vi "Init Cubic Spline + Sine Parameters.vi"(6 "Weighted Fit":T3, 8 "error in (no error)":errorcluster, 9 "Cubic Spline + Sine Options":T1, 10 "Y axis in":dbl[](array[numeric]), 11 "t Axis in":dbl[](array[numeric])) -> (0 "error out":errorcluster, 1 "Cubic Spline + Sine Options":T1, 2 "Initial Parameters":dbl[](array[numeric]), 3 "Weights":dbl[](array[numeric]), 4 "parameter bounds":T2)   [LabVIEW 2021, in "Fits.lvlib"]
uses:
  Fits.lvlib
  Cubic Spline + Sine Options.ctl
  IRF(X)PSED/Fit Weights Type v2.ctl
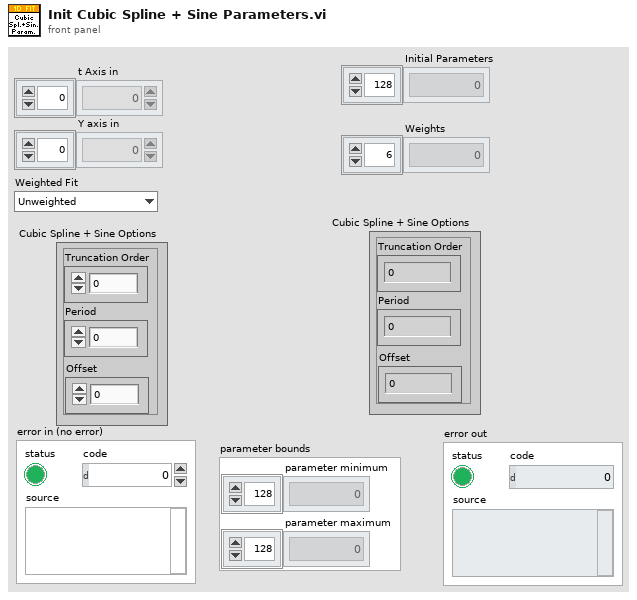
[diagram p1: front panel]
types:
  T1 = typedef "Fits.lvlib/Cubic Spline + Sine Options.ctl" = cluster{"Truncation Order":i32, "Period":dbl, "Offset":dbl}
  T2 = cluster{"parameter minimum":dbl[], "parameter maximum":dbl[]}
  T3 = typedef "Fits.lvlib/Fit Weights Type v2.ctl" = enum16{"Unweighted", "1/Variance (Neyman)", "1/Variance (Pearson)", "Best of All"}
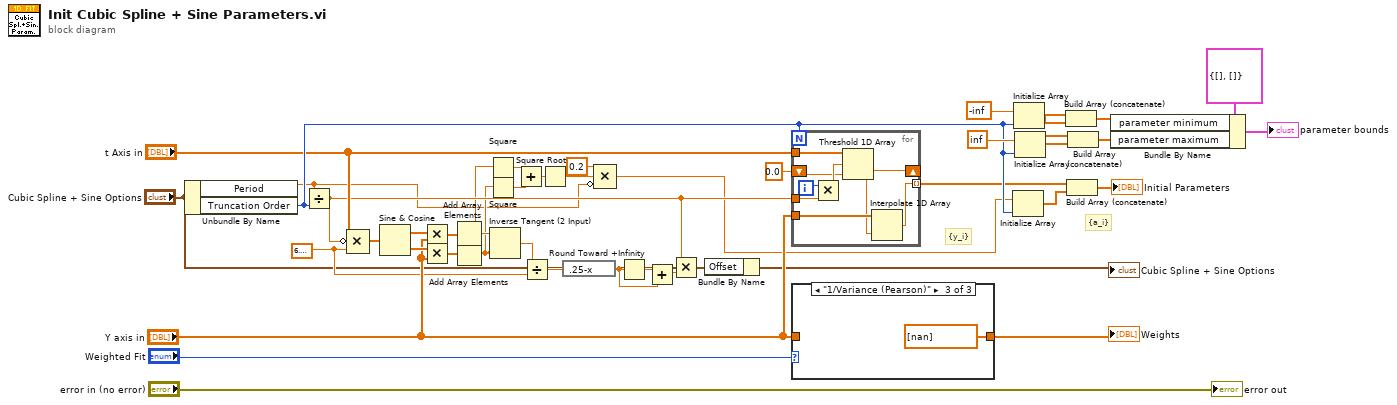
[diagram p0: block diagram]
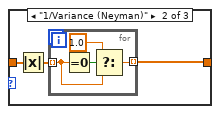
[diagram p3: hidden frame]
diagram:
  w18 = 6.283185307179586
  # "{a_i}"
  # "{y_i}"
  n1 = Unbundle By Name("Cubic Spline + Sine Options") -> ("Period"=w2:dbl, "Truncation Order"=w30:i32)
  n2 = Divide(x=w2, y=w30) -> (x/y=w13:dbl)
  n3 = Compound Arithmetic op=MULTIPLY("t Axis in", invert w13, w18) -> (w25:dbl[])
  n4 = Sine & Cosine(0:w25) -> (1:w23:dbl[], 2:w24:dbl[])
  n5 = Multiply(x=w23, y="Y axis in") -> (x*y=w21:dbl[])
  n6 = Multiply(x=w24, y="Y axis in") -> (x*y=w20:dbl[])
  n7 = Add Array Elements(numeric array=w21) -> (sum=w9:dbl)
  n8 = Add Array Elements(numeric array=w20) -> (sum=w8:dbl)
  n9 = Square(x=w9) -> (x^2=w7:dbl)
  n10 = Square(x=w8) -> (x^2=w6:dbl)
  n11 = Inverse Tangent (2 Input)(1:w8, 2:w9) -> (0:w19:dbl)
  n12 = Add(x=w7, y=w6) -> (x+y=w5:dbl)
  n13 = Divide(x=w19, y=w18) -> (x/y=w17:dbl)
  n14 = Square Root(x=w5) -> (sqrt(x)=w4:dbl)
  n15 = expression code=".25-x"(w17) -> (w15:dbl)
  n16 = Compound Arithmetic op=MULTIPLY(0.2 ("value"), w4, invert w2) -> (w1:dbl)
  n17 = Round Toward +Infinity(x=w15) -> (ceil(x): smallest int >= x=w16:dbl)
  n18 = Add(x=w16, y=w15) -> (x+y=w14:dbl)
  n19 = Multiply(x=w13, y=w14) -> (x*y=w11:dbl)
  n20 = Bundle By Name(cluster="Cubic Spline + Sine Options", "Offset"=w11) -> (→"Cubic Spline + Sine Options":T1)
  n21 = for {
    N: w30 -> [_]
    tunnel: "Y axis in" -> [w50]
    tunnel: [w49] -> w28 mode=indexing
    tunnel: w13 -> [w48]
    tunnel: "t Axis in" -> [w46]
    shift-right: [w43] -> _
    shift-left: 0.0 -> [w44]
    i -> [w47]
    n22 = Multiply(x=w47, y=w48) -> (x*y=w45:dbl)
    n23 = Threshold 1D Array(1:w44, 2:w45, 3:w46) -> (0:w43:dbl)
    n24 = Interpolate 1D Array(1:w43, 2:w50) -> (0:w49:dbl)
  }
  n25 = case shown="\"1/Variance (Pearson)\"" "Weighted Fit" {
    tunnel: "Y axis in" -> [_ w53 _]
    tunnel: [_ w51 dbl[] [nan]] -> w41
    frame "Unweighted", Default {
    }
    frame "1/Variance (Neyman)" {
      n26 = Absolute Value(x=w53) -> (abs(x)=w52:dbl[])
      n27 = for {
        tunnel: w52 -> [w56] mode=indexing
        tunnel: [w54] -> w51 mode=indexing
        n28 = Equal To 0?(x=w56) -> (x = 0?=w57:bool)
        n29 = Select(t=1.0, s=w57, f=w56) -> (s? t:f=w54:dbl)
      }
    }
    frame "1/Variance (Pearson)" {
    }
  }
  "Weights" <- w41
  n30 = Initialize Array(w1, w30) -> (w40:dbl[])
  n31 = Initialize Array(-inf ("element"), w30) -> (w31:dbl[])
  n32 = Initialize Array(inf ("element"), w30) -> (w33:dbl[])
  n33 = Build Array (concatenate)(w31, w31) -> (w27:dbl[])
  n34 = Build Array (concatenate)(w28, w40) -> (→"Initial Parameters":dbl[])
  n35 = Build Array (concatenate)(w33, w33) -> (w35:dbl[])
  n36 = Bundle By Name(cluster=T2 {"parameter minimum"=[], "parameter maximum"=[]} ("parameter bounds"), "parameter minimum"=w27, "parameter maximum"=w35) -> (→"parameter bounds":T2)
  "error out" <- "error in (no error)"
